vi "activationFunction.vi"(11 "input":fxp<+/-,64,32>) -> (3 "activation":fxp<+/-,64,32>)   [LabVIEW 2015]
uses:
  <vilib>/rvi/FXPMathLib/FxpExp/subVIs/nifxpmath_Exp_SimConfig.ctl
  <vilib>/rvi/FXPMathLib/FxpDiv/subVIs/nifxpmath_Div_SimConfig.ctl
  <vilib>/rvi/FXPMathLib/FxpExp/simVIs/DllFxpExpTemp_sub.vi
  <vilib>/rvi/FXPMathLib/FxpDiv/simVIs/DllFxpDivTemp_sub.vi
  <vilib>/rvi/FXPMathLib/FxpMul/XNode/nifxpmath_Multiplier.xnode
  <vilib>/rvi/FXPMathLib/FxpExp/XNode/nifxpmath_Exp.xnode
  <vilib>/rvi/FXPMathLib/FxpAdd/XNode/nifxpmath_Add.xnode
  <vilib>/rvi/FXPMathLib/FxpReciprocal/XNode/nifxpmath_Reciprocal.xnode
  <vilib>/rvi/FXPMathLib/FxpDiv/XNode/nifxpmath_Div.xnode
  <vilib>/rvi/FXPMathLib/sim/FxpSim.dll
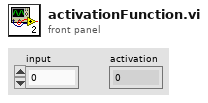
[diagram p1: front panel]
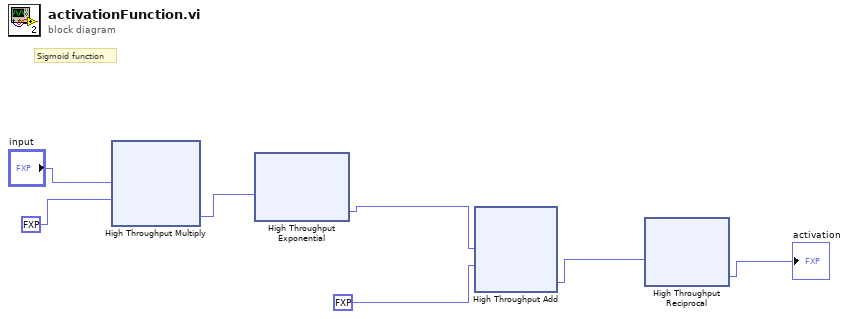
[diagram p0: block diagram]
diagram:
  # "Sigmoid function"
  n1 = xnode "High Throughput Multiply"("x"="input", "y"=fxp<+/-,1,1> -1.0) -> ("x*y"=w7:fxp<+/-,16,1>)
  n2 = xnode "High Throughput Exponential"("x"=w7) -> ("exp(x)"=w6:fxp<+,16,2>)
  n3 = xnode "High Throughput Add"("x"=w6, "y"=fxp<+,1,1> 1.0) -> ("x+y"=w4:fxp<+,17,3>)
  n4 = xnode "High Throughput Reciprocal"("x"=w4) -> ("1/x"=→"activation":fxp<+,17,14>)
